vi "hilbert fir.vi"(4 "x(n)":fxp<+/-,20,4>) -> (1 "y(n)":fxp<+/-,20,4>)   [LabVIEW 2014]
uses:
  <vilib>/rvi/FXPMathLib/FxpConvert/subVIs/nifxpmath_Convert_SimConfig.ctl
  <vilib>/fxp/LVFixedPointQuantizationPolicyTypeDef.ctl
  <vilib>/fxp/LVFixedPointOverflowPolicyTypeDef.ctl
  <vilib>/rvi/FXPMathLib/FxpConvert/simVIs/DllFxpConvertTemp_sub.vi
  <vilib>/rvi/FXPMathLib/FxpSub/XNode/nifxpmath_Sub.xnode
  <vilib>/rvi/FXPMathLib/FxpMul/XNode/nifxpmath_Multiplier.xnode
  <vilib>/rvi/FXPMathLib/FxpAdd/XNode/nifxpmath_Add.xnode
  <vilib>/rvi/FXPMathLib/FxpConvert/XNode/nifxpmath_Convert.xnode
  <vilib>/rvi/FXPMathLib/sim/FxpSim.dll
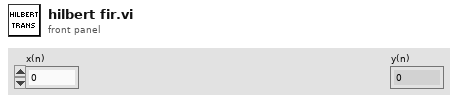
[diagram p1: front panel]
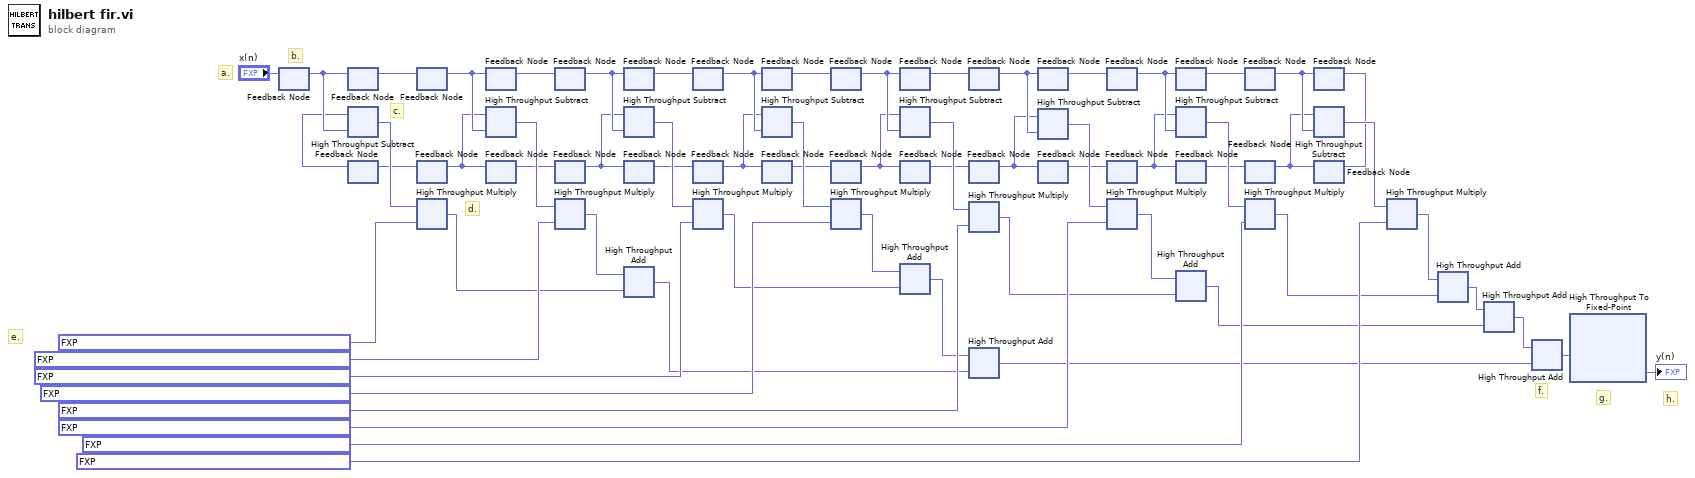
[diagram p0: block diagram]
diagram:
  # "h."
  # "g."
  # "f."
  # "e."
  # "d."
  # "c."
  # "b."
  # "a."
  n1 = feedback #1() -> (w33:fxp<+/-,20,4>)  [unwired: 1 in]
  n2 = feedback-in #1("x(n)") -> ()
  n3 = feedback #2() -> (w32:fxp<+/-,20,4>)  [unwired: 1 in]
  n4 = feedback-in #2(w33) -> ()
  n5 = feedback #3() -> (w3:fxp<+/-,20,4>)  [unwired: 1 in]
  n6 = xnode "High Throughput Subtract"("x"=w3, "y"=w33) -> ("x-y"=w64:fxp<+/-,21,5>)
  n7 = feedback #4() -> (w31:fxp<+/-,20,4>)  [unwired: 1 in]
  n8 = feedback-in #4(w32) -> ()
  n9 = feedback #5() -> (w4:fxp<+/-,20,4>)  [unwired: 1 in]
  n10 = feedback-in #3(w4) -> ()
  n11 = xnode ("High Throughput Multiply")("x"=w64, "y"=fxp<+,41,-7> 0.004215989128468323 ("Numeric")) -> ("x*y"=w47:fxp<+/-,62,-2>)
  n12 = feedback #6() -> (w30:fxp<+/-,20,4>)  [unwired: 1 in]
  n13 = feedback-in #6(w31) -> ()
  n14 = feedback #7() -> (w5:fxp<+/-,20,4>)  [unwired: 1 in]
  n15 = feedback-in #5(w5) -> ()
  n16 = xnode "High Throughput Subtract"("x"=w5, "y"=w31) -> ("x-y"=w61:fxp<+/-,21,5>)
  n17 = feedback #8() -> (w29:fxp<+/-,20,4>)  [unwired: 1 in]
  n18 = feedback-in #8(w30) -> ()
  n19 = feedback #9() -> (w6:fxp<+/-,20,4>)  [unwired: 1 in]
  n20 = feedback-in #7(w6) -> ()
  n21 = xnode ("High Throughput Multiply")("x"=w61, "y"=fxp<+,45,-6> 0.009298295547623958 ("Numeric")) -> ("x*y"=w48:fxp<+/-,64,-1>)
  n22 = feedback #10() -> (w28:fxp<+/-,20,4>)  [unwired: 1 in]
  n23 = feedback-in #10(w29) -> ()
  n24 = feedback #11() -> (w7:fxp<+/-,20,4>)  [unwired: 1 in]
  n25 = feedback-in #9(w7) -> ()
  n26 = xnode "High Throughput Subtract"("x"=w7, "y"=w29) -> ("x-y"=w59:fxp<+/-,21,5>)
  n27 = xnode ("High Throughput Add")("x"=w48, "y"=w47) -> ("x+y"=w39:fxp<+/-,64,0>)
  n28 = feedback #12() -> (w27:fxp<+/-,20,4>)  [unwired: 1 in]
  n29 = feedback-in #12(w28) -> ()
  n30 = feedback #13() -> (w8:fxp<+/-,20,4>)  [unwired: 1 in]
  n31 = feedback-in #11(w8) -> ()
  n32 = xnode ("High Throughput Multiply")("x"=w59, "y"=fxp<+,45,-5> 0.018853050583680364 ("Numeric")) -> ("x*y"=w45:fxp<+/-,64,0>)
  n33 = feedback #14() -> (w26:fxp<+/-,20,4>)  [unwired: 1 in]
  n34 = feedback-in #14(w27) -> ()
  n35 = feedback #15() -> (w9:fxp<+/-,20,4>)  [unwired: 1 in]
  n36 = feedback-in #13(w9) -> ()
  n37 = xnode "High Throughput Subtract"("x"=w9, "y"=w27) -> ("x-y"=w53:fxp<+/-,21,5>)
  n38 = feedback #16() -> (w25:fxp<+/-,20,4>)  [unwired: 1 in]
  n39 = feedback-in #16(w26) -> ()
  n40 = feedback #17() -> (w10:fxp<+/-,20,4>)  [unwired: 1 in]
  n41 = feedback-in #15(w10) -> ()
  n42 = xnode ("High Throughput Multiply")("x"=w53, "y"=fxp<+,45,-4> 0.03441454817865086 ("Numeric")) -> ("x*y"=w46:fxp<+/-,64,1>)
  n43 = feedback #18() -> (w24:fxp<+/-,20,4>)  [unwired: 1 in]
  n44 = feedback-in #18(w25) -> ()
  n45 = feedback #19() -> (w11:fxp<+/-,20,4>)  [unwired: 1 in]
  n46 = feedback-in #17(w11) -> ()
  n47 = xnode "High Throughput Subtract"("x"=w11, "y"=w25) -> ("x-y"=w52:fxp<+/-,21,5>)
  n48 = xnode ("High Throughput Add")("x"=w46, "y"=w45) -> ("x+y"=w40:fxp<+/-,64,2>)
  n49 = feedback #20() -> (w23:fxp<+/-,20,4>)  [unwired: 1 in]
  n50 = feedback-in #20(w24) -> ()
  n51 = feedback #21() -> (w12:fxp<+/-,20,4>)  [unwired: 1 in]
  n52 = feedback-in #19(w12) -> ()
  n53 = xnode ("High Throughput Multiply")("x"=w52, "y"=fxp<+,45,-4> 0.05956444175878062 ("Numeric")) -> ("x*y"=w43:fxp<+/-,64,1>)
  n54 = xnode ("High Throughput Add")("x"=w40, "y"=w39) -> ("x+y"=w35:fxp<+/-,64,3>)
  n55 = feedback #22() -> (w22:fxp<+/-,20,4>)  [unwired: 1 in]
  n56 = feedback-in #22(w23) -> ()
  n57 = feedback #23() -> (w13:fxp<+/-,20,4>)  [unwired: 1 in]
  n58 = feedback-in #21(w13) -> ()
  n59 = xnode "High Throughput Subtract"("x"=w13, "y"=w23) -> ("x-y"=w51:fxp<+/-,21,5>)
  n60 = feedback #24() -> (w21:fxp<+/-,20,4>)  [unwired: 1 in]
  n61 = feedback-in #24(w22) -> ()
  n62 = feedback #25() -> (w14:fxp<+/-,20,4>)  [unwired: 1 in]
  n63 = feedback-in #23(w14) -> ()
  n64 = xnode ("High Throughput Multiply")("x"=w51, "y"=fxp<+,45,-3> 0.10304544022280027 ("Numeric")) -> ("x*y"=w44:fxp<+/-,64,2>)
  n65 = feedback #26() -> (w20:fxp<+/-,20,4>)  [unwired: 1 in]
  n66 = feedback-in #26(w21) -> ()
  n67 = feedback #27() -> (w15:fxp<+/-,20,4>)  [unwired: 1 in]
  n68 = feedback-in #25(w15) -> ()
  n69 = xnode "High Throughput Subtract"("x"=w15, "y"=w21) -> ("x-y"=w50:fxp<+/-,21,5>)
  n70 = xnode ("High Throughput Add")("x"=w44, "y"=w43) -> ("x+y"=w37:fxp<+/-,64,3>)
  n71 = feedback #28() -> (w19:fxp<+/-,20,4>)  [unwired: 1 in]
  n72 = feedback-in #28(w20) -> ()
  n73 = feedback #29() -> (w16:fxp<+/-,20,4>)  [unwired: 1 in]
  n74 = feedback-in #27(w16) -> ()
  n75 = xnode ("High Throughput Multiply")("x"=w50, "y"=fxp<+,45,-2> 0.1968363540916016 ("Numeric")) -> ("x*y"=w41:fxp<+/-,64,3>)
  n76 = feedback #30() -> (w18:fxp<+/-,20,4>)  [unwired: 1 in]
  n77 = feedback-in #30(w19) -> ()
  n78 = feedback #31() -> (w17:fxp<+/-,20,4>)  [unwired: 1 in]
  n79 = feedback-in #29(w17) -> ()
  n80 = xnode "High Throughput Subtract"("x"=w17, "y"=w19) -> ("x-y"=w49:fxp<+/-,21,5>)
  n81 = feedback-in #31(w18) -> ()
  n82 = xnode ("High Throughput Multiply")("x"=w49, "y"=fxp<+,45,0> 0.6313558292569041 ("Numeric")) -> ("x*y"=w42:fxp<+/-,64,5>)
  n83 = xnode ("High Throughput Add")("x"=w42, "y"=w41) -> ("x+y"=w38:fxp<+/-,64,6>)
  n84 = xnode ("High Throughput Add")("x"=w38, "y"=w37) -> ("x+y"=w36:fxp<+/-,64,7>)
  n85 = xnode ("High Throughput Add")("x"=w36, "y"=w35) -> ("x+y"=w2:fxp<+/-,64,8>)
  n86 = xnode "High Throughput To Fixed-Point"("x"=w2) -> ("y"=→"y(n)":fxp<+/-,20,4>)
